vi "initPressure_topLvl.vi"(8 "error in":errorcluster, 11 "Pressure box control in":T1={"Pressure box COM"="", "pressure box type"=enum."Neuromatics", "High pos pressure (mBar)"=200.0, "Low pos pressure (mBar)"=80.0, "Vacuum pressure (mBar)"=-40.0, "calibration"=enum."PA_vacPump"}) -> (0 "error out":errorcluster, 3 "Pressure box control out":T1={"Pressure box COM"="", "pressure box type"=enum."Neuromatics", "High pos pressure (mBar)"=200.0, "Low pos pressure (mBar)"=80.0, "Vacuum pressure (mBar)"=-40.0, "calibration"=enum."PA_vacPump"})   [LabVIEW 2015]
uses:
  <vilib>/Instr/_visa.llb/VISA Configure Serial Port (Instr).vi
  controls/pressure_box_type.ctl
  controls/pressure_box_control.ctl
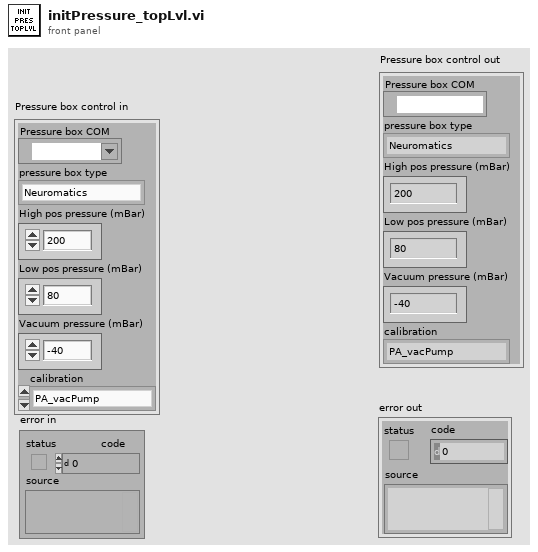
[diagram p1: front panel]
types:
  T1 = typedef "pressure_box_control.ctl" = cluster{"Pressure box COM":refnum<visa-resource-name>, "pressure box type":T2, "High pos pressure (mBar)":dbl, "Low pos pressure (mBar)":dbl, "Vacuum pressure (mBar)":dbl, "calibration":enum16{"PA_vacPump", "PA_venturi", "Neuromatics", "ilyaRig", "mightenRig"}}
  T2 = typedef "pressure_box_type.ctl" = enum16{"Neuromatics", "ProportionAir", "Demo box", "N-ProportionAir"}
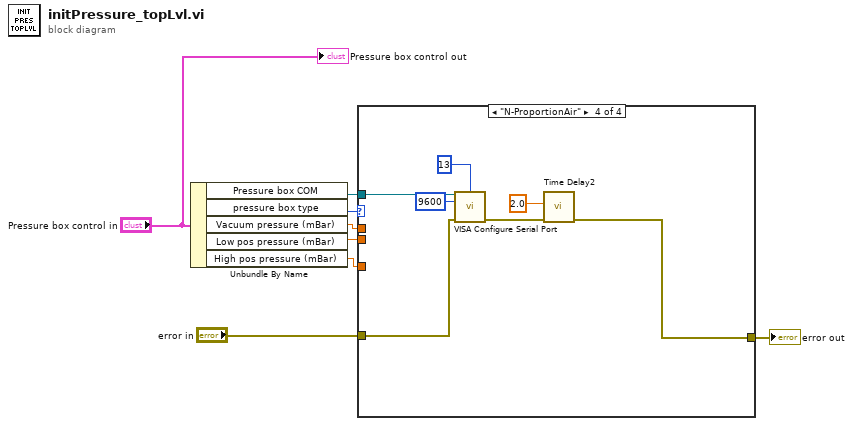
[diagram p0: block diagram]
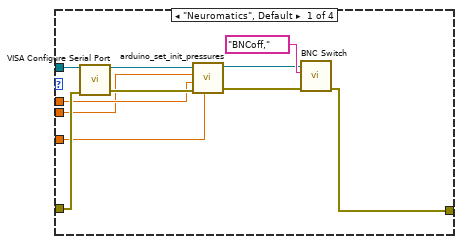
[diagram p2: hidden frame]
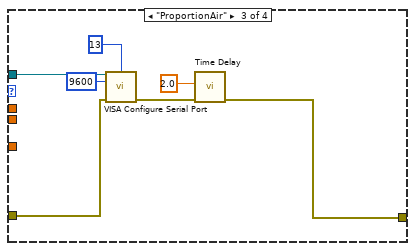
[diagram p4: hidden frame]
diagram:
  n1 = Unbundle By Name("Pressure box control in") -> ("Pressure box COM"=w7:refnum<visa-resource-name>, "pressure box type"=w8:T2, "Vacuum pressure (mBar)"=w3:dbl, "Low pos pressure (mBar)"=w2:dbl, "High pos pressure (mBar)"=w1:dbl)
  n2 = case shown="\"N-ProportionAir\"" w8 {
    tunnel: w7 -> [w18 _ w25 w32]
    tunnel: [w9 w20 w23 w30] -> w6
    tunnel: "error in" -> [w13 w20 w22 w29]
    tunnel: w3 -> [w12 _ _ _]
    tunnel: w2 -> [w11 _ _ _]
    tunnel: w1 -> [w10 _ _ _]
    frame "Neuromatics", Default {
      n3 = call-poly "VISA Configure Serial Port"("VISA resource name"=w18, "error in (no error)"=w13) -> ("VISA resource name out"=w17:refnum<visa-resource-name>, "error out"=w14:errorcluster)  [unwired: 12 in]
      n4 = call "arduino_set_init_pressures.vi"("High P"=w10, "error in"=w14, "Suction"=w12, "Low P"=w11, "Pressure Box COM in"=w17) -> ("error out"=w15:errorcluster, "Pressure Box COM out"=w16:refnum<visa-resource-name>)  [unwired: 5 in]
      n5 = call "BNC Switch.vi"("error in"=w15, "BNC command"="BNCoff,", "Pressure Box COM"=w16) -> ("error out"=w9:errorcluster)  [unwired: 6 in, 2 out]
    }
    frame "Demo box" {
    }
    frame "ProportionAir" {
      n6 = call-poly "VISA Configure Serial Port"("VISA resource name"=w25, "termination char\n(0xA = '\\n' = LF)"=u8 13 ("termination char\n(0xA = '\\n' = LF)"), "baud rate (9600)"=u32 9600, "error in (no error)"=w22) -> ("error out"=w24:errorcluster)  [unwired: 10 in, 1 out]
      n7 = call "Time Delay"("error in (no error)"=w24, "Delay Time (s)"=2.0) -> ("error out"=w23:errorcluster)  [unwired: 9 in]
    }
    frame "N-ProportionAir" {
      n8 = call-poly "VISA Configure Serial Port"("VISA resource name"=w32, "termination char\n(0xA = '\\n' = LF)"=u8 13 ("termination char\n(0xA = '\\n' = LF)"), "baud rate (9600)"=u32 9600, "error in (no error)"=w29) -> ("error out"=w31:errorcluster)  [unwired: 10 in, 1 out]
      n9 = call "Time Delay2"("error in (no error)"=w31, "Delay Time (s)"=2.0) -> ("error out"=w30:errorcluster)  [unwired: 9 in]
    }
  }
  "error out" <- w6
  "Pressure box control out" <- "Pressure box control in"
